vi "trackerhandle.vi"(3 "error in":errorcluster, 4 "action":enum16{"get", "set"}(ring), 5 "input Cluster":T1={"ROI1"=0, "Rmax (pix)"=32, "RminZ (pix)"=0, "LUTs"=[], "use trace"=FALSE, "angular pixel\n coverage factor"=0.0, "radial pixel\n coverage factor"=0.0}) -> (0 "error out":errorcluster, 2 "output Cluster":T1={"ROI1"=0, "Rmax (pix)"=32, "RminZ (pix)"=0, "LUTs"=[], "use trace"=FALSE, "angular pixel\n coverage factor"=0.0, "radial pixel\n coverage factor"=0.0})   [LabVIEW 2011, in "OfflineTracker.lvlib"]
uses:
  OfflineTracker.lvlib
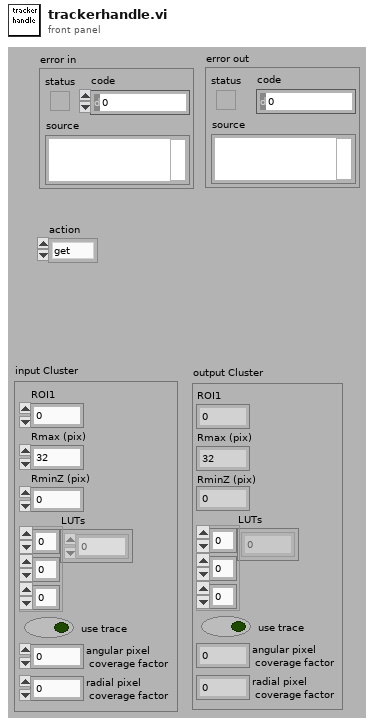
[diagram p1: front panel]
types:
  T1 = cluster{"ROI1":i32, "Rmax (pix)":i32, "RminZ (pix)":i32, "LUTs":dbl[][][], "use trace":bool, "angular pixel\n coverage factor":dbl, "radial pixel\n coverage factor":dbl}
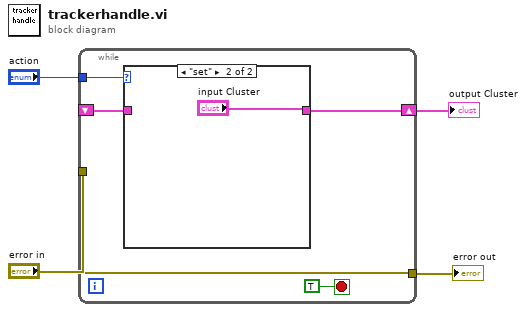
[diagram p0: block diagram]
diagram:
  n1 = while {
    tunnel: "error in" -> [w8]
    tunnel: [w8] -> w2
    shift-right: [w5] -> w1
    shift-left: _ -> [w7]
    tunnel: "action" -> [w6]
    stop <- TRUE ("stop") stop-if-true
    n2 = case shown="\"set\"" w6 {
      tunnel: w7 -> [w10 _]
      tunnel: [w10 "input Cluster"] -> w5
      frame "get" {
      }
      frame "set" {
      }
    }
  }
  "error out" <- w2
  "output Cluster" <- w1
